vi "nivsfpga_AddDmaFifoToProject.vi"(6 "number of elements":u32, 8 "error in (no error)":errorcluster, 9 "type":T1, 10 "name":string, 11 "FPGA Target ref in":refnum<vi>) -> (0 "error out":errorcluster, 2 "DMA FIFO ref":refnum<vi>, 3 "reference out":refnum<vi>)   [LabVIEW 2010]
uses:
  <vilib>/rvi/ClientSDK/Core/Script/Container/Item/Public/niFpgaContainerItemScriptType.ctl
  <vilib>/rvi/ClientSDK/Core/Script/Container/Item/Public/niFpgaContainerItemScriptDataType.ctl
  <vilib>/rvi/ClientSDK/Core/Script/Container/Item/Public/niFpgaContainerItemScriptImplementation.ctl
  <vilib>/rvi/ClientSDK/Core/Script/Container/Item/Public/niFpgaContainerItemScriptArbitration.ctl
  <vilib>/fxp/LVFixedPointRepBitsTypeDef.ctl
  <vilib>/rvi/ClientSDK/Core/Script/Container/Item/Public/niFpgaContainerItemScriptContainerType.ctl
  <vilib>/rvi/ClientSDK/Core/Script/Container/Item/Private/Create_ProjectItem.vi
  <vilib>/rvi/ClientSDK/Core/Script/Container/Item/Private/SetValue_NumberOfElements.vi
  <vilib>/rvi/ClientSDK/Core/Script/Container/Item/Private/SetValue_DataType.vi
  <vilib>/rvi/ClientSDK/Core/Script/Container/Item/Private/SetValue_ArbitrationForReadAndWrite.vi
  <vilib>/rvi/ClientSDK/Core/Script/Container/Item/Private/SetValue_Implementation.vi
  <vilib>/rvi/ClientSDK/Core/Script/Container/Item/Private/SetValue_Type.vi
  <vilib>/rvi/ClientSDK/Core/Script/Container/Item/Private/niFpgaContainerItemScript.lvclass
  <vilib>/Utility/VariantDataType/VariantType.lvlib
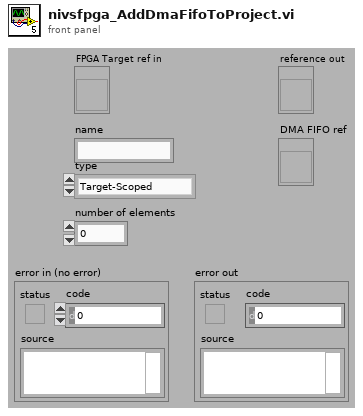
[diagram p1: front panel]
types:
  T1 = typedef "niFpgaContainerItemScriptType.ctl" = enum16{"Target-Scoped", "Host to Target - DMA", "Target to Host - DMA", "Peer to Peer Reader", "Peer to Peer Writer", "Bidirectional"}
  T2 = typedef "niFpgaContainerItemScriptDataType.ctl" = enum32{"Boolean", "I8", "I16", "I32", "I64", "U8", "U16", "U32", "U64", "FXP", "CustomControl"}
  T3 = typedef "niFpgaContainerItemScriptImplementation.ctl" = enum16{"Flip-Flops", "Look-Up Table", "Block Memory", "DRAM"}
  T4 = typedef "niFpgaContainerItemScriptArbitration.ctl" = enum16{"Always Arbitrate", "Arbitrate if Multiple Requestors Only", "Never Arbitrate"}
  T5 = cluster{"name":string, "type":T1, "number of elements":u32, "data type":T2, "implementation":T3, "read arbitration":T4, "write arbitration":T4}
  T6 = typedef "niFpgaContainerItemScriptContainerType.ctl" = enum16{"FIFO", "Memory", "Register"}
  T7 = typedef "LVFixedPointRepBitsTypeDef.ctl" = cluster{"Signed":bool, "Word Length":u32, "Integer Word Length":i32}
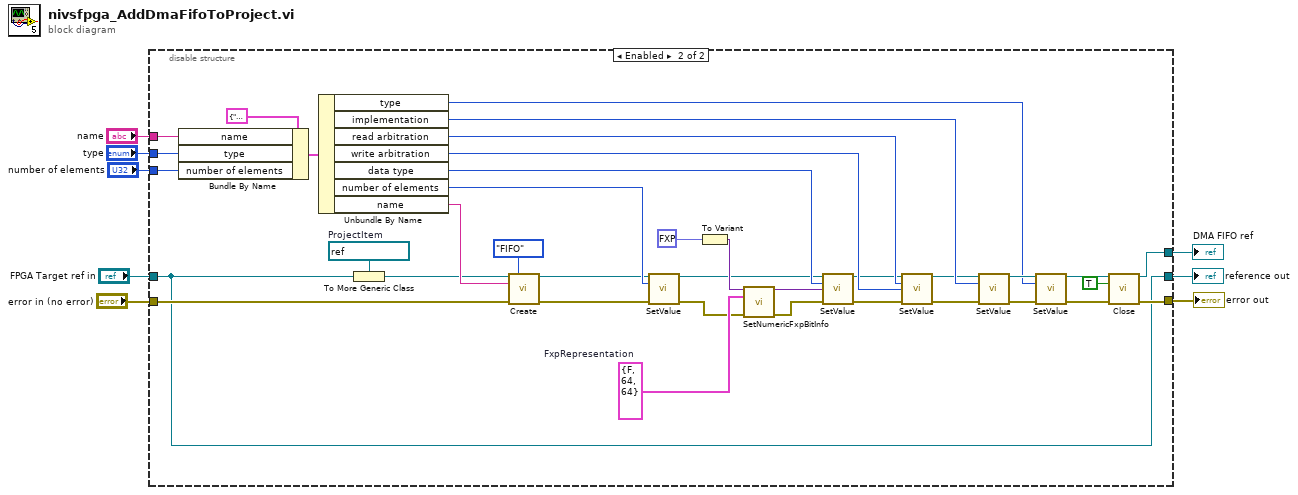
[diagram p0: block diagram]
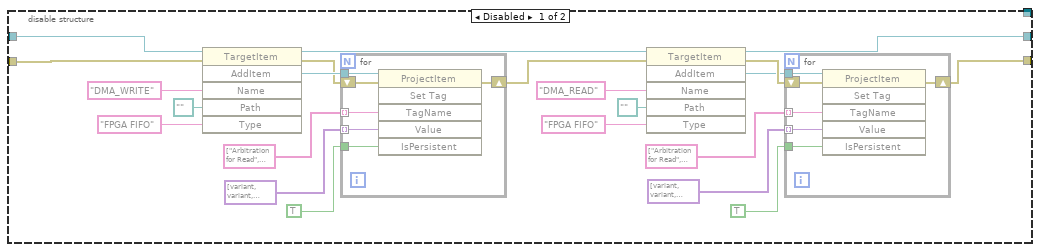
[diagram p2: hidden frame]
diagram:
  n1 = disable-structure shown="Enabled" {
    disable-tunnel: "error in (no error)" -> [w30 w54]
    disable-tunnel: "FPGA Target ref in" -> [w29 w49]
    disable-tunnel: [w28 w49] -> w6
    disable-tunnel: [w27 w50] -> w5
    disable-tunnel: "number of elements" -> [_ w53]
    disable-tunnel: "type" -> [_ w52]
    disable-tunnel: "name" -> [_ w51]
    disable-tunnel: [_ w43] -> w1
    frame Disabled {
      n2 = invoke class="TargetItem" method="AddItem"(reference=w29, error in=w30, "Name"="DMA_WRITE", "Path"=path "", "Type"="FPGA FIFO") -> (reference out=w11:refnum<vi>, error out=w20:errorcluster, "AddItem"=w23:refnum<vi>)  [unwired: 1 in, 3 out]
      n3 = for {
        tunnel: w23 -> [w42]
        tunnel: string[] ["Arbitration for Read", "Arbitration for Write", "Data Type", "Disable on Overflow/Underflow", "DMA Channel", "fifo.configuration", "fifo.configured", "fifo.projectItemValid", "fifo.valid", "fifo.version", "FPGA.PersistentID", "FXP Delta", "FXP Int Word Length", "FXP Maximum", "FXP Minimum", "FXP Signed", "FXP Word Length", "Implementation", "Local", "Number of Elements", "Type"] ("Tag:Get Names") -> [w41] mode=indexing
        tunnel: variant[] [variant(u32 1), variant(u32 1), variant(u32 8), variant(bool FALSE), variant(u32 0), variant(string "\"NumberOfElements=21;DataType=8;Type=1;ReadArbs=Arbitrate if Multiple Requestors Only;WriteArbs=Arbitrate if Multiple Requestors Only;Implementation=2;DMA_WRITE;FxpWordLength=64;FxpIntWordLength=64;FxpSigned=FALSE;FxpMin=0.000000;FxpMax=18446744073709551600.000000;FxpDelta=1.000000\""), variant(bool TRUE), variant(bool TRUE), variant(bool TRUE), variant(i32 9), variant(string "{6DD9639D-8794-446C-84EA-1599FD403AE2}"), variant(string "1.0000000000000000000000000000000000000000000000000000000E+0"), variant(i32 64), variant(string "1.8446744073709552000000000000000000000000000000000000000E+19"), variant(string "0.0000000000000000000000000000000000000000000000000000000E+0"), variant(bool FALSE), variant(u32 64), variant(u32 2), variant(bool FALSE), variant(u32 21), variant(u32 1)] ("Array") -> [w40] mode=indexing
        tunnel: TRUE ("IsPersistent") -> [w39]
        shift-right: [w37] -> w12
        shift-left: w20 -> [w38]
        n4 = invoke class="ProjectItem" method="Set Tag"(reference=w42, error in=w38, "TagName"=w41, "Value"=w40, "IsPersistent"=w39) -> (error out=w37:errorcluster)  [unwired: 1 in, 5 out]
      }
      n5 = invoke class="TargetItem" method="AddItem"(reference=w11, error in=w12, "Name"="DMA_READ", "Path"=path "", "Type"="FPGA FIFO") -> (reference out=w28:refnum<vi>, error out=w17:errorcluster, "AddItem"=w16:refnum<vi>)  [unwired: 1 in, 3 out]
      n6 = for {
        tunnel: w16 -> [w36]
        tunnel: string[] ["Arbitration for Read", "Arbitration for Write", "Data Type", "Disable on Overflow/Underflow", "DMA Channel", "fifo.configuration", "fifo.configured", "fifo.projectItemValid", "fifo.valid", "fifo.version", "FPGA.PersistentID", "FXP Delta", "FXP Int Word Length", "FXP Maximum", "FXP Minimum", "FXP Signed", "FXP Word Length", "Implementation", "Local", "Number of Elements", "Type"] ("Tag:Get Names") -> [w35] mode=indexing
        tunnel: variant[] [variant(u32 1), variant(u32 1), variant(u32 8), variant(bool FALSE), variant(u32 0), variant(string "\"NumberOfElements=15;DataType=8;Type=2;ReadArbs=Arbitrate if Multiple Requestors Only;WriteArbs=Arbitrate if Multiple Requestors Only;Implementation=2;DMA_READ;FxpWordLength=64;FxpIntWordLength=64;FxpSigned=FALSE;FxpMin=0.000000;FxpMax=18446744073709551600.000000;FxpDelta=1.000000\""), variant(bool TRUE), variant(bool TRUE), variant(bool TRUE), variant(i32 9), variant(string "{E9CF0955-443A-4CAF-B305-16D3E2D85672}"), variant(string "1.0000000000000000000000000000000000000000000000000000000E+0"), variant(i32 64), variant(string "1.8446744073709552000000000000000000000000000000000000000E+19"), variant(string "0.0000000000000000000000000000000000000000000000000000000E+0"), variant(bool FALSE), variant(u32 64), variant(u32 2), variant(bool FALSE), variant(u32 15), variant(u32 2)] ("Array") -> [w34] mode=indexing
        tunnel: TRUE ("IsPersistent") -> [w33]
        shift-right: [w31] -> w27
        shift-left: w17 -> [w32]
        n7 = invoke class="ProjectItem" method="Set Tag"(reference=w36, error in=w32, "TagName"=w35, "Value"=w34, "IsPersistent"=w33) -> (error out=w31:errorcluster)  [unwired: 1 in, 5 out]
      }
    }
    frame Enabled {
      w76 = T7 {"Signed"=FALSE, "Word Length"=64, "Integer Word Length"=64}  # FxpRepresentation
      w79 = refnum<vi> refnum  # ProjectItem
      n8 = Bundle By Name(cluster=T5 {"name"="DMA_READ", "type"=enum."Target to Host - DMA", "number of elements"=15, "data type"=enum."U64", "implementation"=enum."Block Memory", "read arbitration"=enum."Arbitrate if Multiple Requestors Only", "write arbitration"=enum."Arbitrate if Multiple Requestors Only"} ("FIFO test configuration"), "name"=w51, "type"=w52, "number of elements"=w53) -> (w77:T5)
      n9 = Unbundle By Name(w77) -> ("type"=w44:T1, "implementation"=w73:T3, "read arbitration"=w72:T4, "write arbitration"=w71:T4, "data type"=w70:T2, "number of elements"=w69:u32, "name"=w68:string)
      n10 = To More Generic Class(target class=w79, reference=w49) -> (generic class reference=w55:refnum<vi>)
      n11 = call-poly <vilib>:"Create.vi"("parent item"=w55, "container type"=niFpgaContainerItemScriptContainerType."FIFO", "name"=w68, "error in (no error)"=w54) -> ("container out"=w57:refnum<class "niFpgaContainerItemScript.lvclass">, "error out"=w58:errorcluster)  [unwired: 10 in]
      n12 = call-poly <vilib>:"SetValue.vi"("container in"=w57, "number of elements"=w69, "error in (no error)"=w58) -> ("container out"=w59:refnum<class "niFpgaContainerItemScript.lvclass">, "error out"=w60:errorcluster)  [unwired: 11 in]
      n13 = To Variant(anything=fxp<+,1,1> 0.0) -> (Variant=w75:variant)
      n14 = call <vilib>:"SetNumericFxpBitInfo.vi"("Variant"=w75, "FxpRepresentation"=w76, "error in (no error)"=w60) -> ("Modified Variant"=w62:variant, "error out"=w61:errorcluster)  [unwired: 11 in]
      n15 = call-poly <vilib>:"SetValue.vi"("container in"=w59, "data type"=w70, "type descriptor"=w62, "error in (no error)"=w61) -> ("container out"=w63:refnum<class "niFpgaContainerItemScript.lvclass">, "error out"=w64:errorcluster)  [unwired: 10 in]
      n16 = call-poly <vilib>:"SetValue.vi"("container in"=w63, "read arbitration"=w72, "write arbitration"=w71, "error in (no error)"=w64) -> ("container out"=w65:refnum<class "niFpgaContainerItemScript.lvclass">, "error out"=w66:errorcluster)  [unwired: 10 in]
      n17 = call-poly <vilib>:"SetValue.vi"("containter in"=w65, "implementation"=w73, "error in (no error)"=w66) -> ("container out"=w45:refnum<class "niFpgaContainerItemScript.lvclass">, "error out"=w48:errorcluster)  [unwired: 11 in]
      n18 = call-poly <vilib>:"SetValue.vi"("container in"=w45, "type"=w44, "error in (no error)"=w48) -> ("container out"=w46:refnum<class "niFpgaContainerItemScript.lvclass">, "error out"=w47:errorcluster)  [unwired: 11 in]
      n19 = call <vilib>:"Close.vi"("container in"=w46, "return ref"=TRUE, "error in (no error)"=w47) -> ("project item ref"=w43:refnum<vi>, "error out"=w50:errorcluster)  [unwired: 10 in, 1 out]
    }
  }
  "reference out" <- w6
  "error out" <- w5
  "DMA FIFO ref" <- w1
